vi "Globals.vi"() -> ()   [LabVIEW 2015, in "SB SubVIs.lvlib"]
uses:
  SB SubVIs.lvlib
  Type Defs/UI Refs.ctl
  Type Defs/Dashboard.ctl
  Type Defs/Square Cluster.ctl
  Square/Square.lvclass
  Type Defs/SB Type Defs.lvlib
panel:
  out "Attack Q":refnum<queue>
  in  "Map DVR":refnum<data-value>
  in  "Mouse Down":cluster{"X":dbl, "Y":dbl}
  in  "Pan":cluster{"Horizontal":dbl, "Vertical":dbl}
  out "Exit":bool
  out "Running":bool
  in  "UI Refs":T1
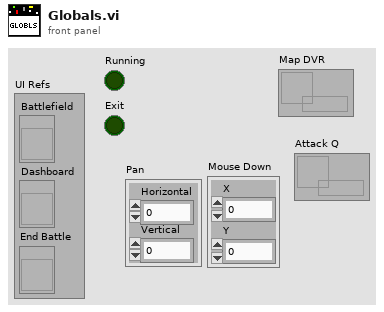
[diagram p1: front panel]
types:
  T1 = typedef "SB Type Defs.lvlib/UI Refs.ctl" = cluster{"Battlefield":refnum<vi>, "Dashboard":refnum<vi>, "End Battle":refnum<vi>}
diagram:
